vi "Midi_SerialComm.vi"(6 "CtrlC":bool, 8 "error in (no error)":errorcluster, 9 "wait for":string, 10 "To send":string, 11 "hub":string) -> (0 "error out":errorcluster, 2 "read":string)   [LabVIEW 2022 SP3]
panel:
  out "guess":string
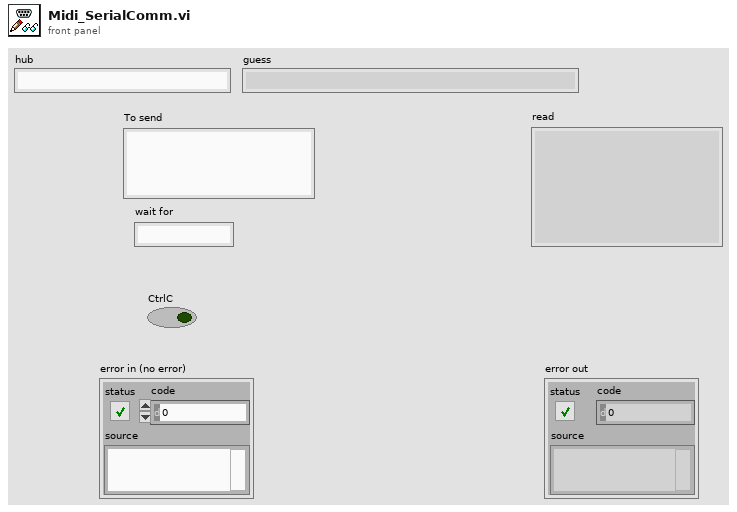
[diagram p1: front panel]
types:
  T1 = typedef "PythonCtrl.ctl" = cluster{"session":refnum<k35>, "PyPath":path, "Processor":T2, "Port":string, "version":string}
  T2 = typedef "Processors.ctl" = enum16{"SPIKE", "Pi", "Pi_ssh", "OpenMV", "Dunio"}
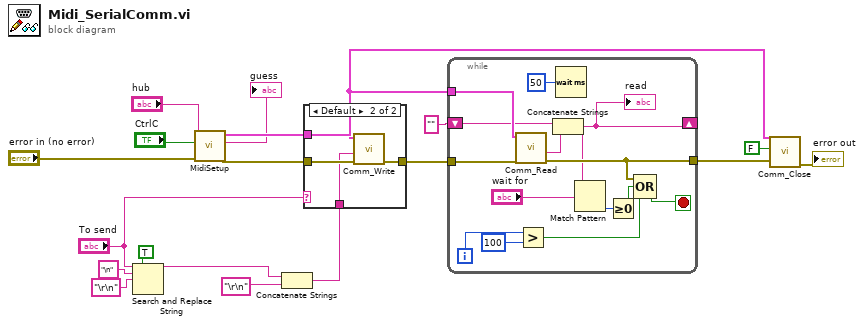
[diagram p0: block diagram]
diagram:
  n1 = Search and Replace String(replace all?=TRUE ("replace all? (F)"), input string="To send", search string="\n" ("function name"), replace string="\r\n" ("function name")) -> (result string=w6:string)  [unwired: 4 in, 3 out]
  n2 = call "MidiSetup.vi"("error in (no error)"="error in (no error)", "CtrlC"="CtrlC", "hub"="hub") -> ("error out"=w17:errorcluster, "guess"=→"guess":string, "Python"=w15:T1)  [unwired: 6 in]
  n3 = Concatenate Strings(w6, "\r\n" ("function name")) -> (w11:string)
  n4 = case shown="Default" "To send" {
    tunnel: w17 -> [w19 w23]
    tunnel: [w19 w22] -> w16
    tunnel: w15 -> [_ w21]
    tunnel: w11 -> [_ w20]
    frame "" {
    }
    frame Default {
      n5 = call "Comm_Write.vi"("error in (no error)"=w23, "Text to write"=w20, "Python"=w21) -> ("error out"=w22:errorcluster)  [unwired: 7 in, 1 out]
    }
  }
  n6 = while {
    tunnel: w16 -> [w37]
    tunnel: w15 -> [w36]
    tunnel: [w30] -> w14
    shift-right: [w27] -> _
    shift-left: "" -> [w34]
    i -> [w26]
    stop <- w29 stop-if-true
    n7 = call "Comm_Read.vi"("error in (no error)"=w37, "Python"=w36) -> ("error out"=w30:errorcluster, "Text read"=w35:string)  [unwired: 8 in]
    n8 = Greater?(x=w26, y=100) -> (0:w24:bool)
    n9 = Concatenate Strings(w34, w35) -> (w27:string)
    "read" <- w27
    n10 = Wait (ms)(milliseconds to wait=u32 50) -> ()  [unwired: 1 out]
    n11 = Match Pattern(string=w27, regular expression="wait for") -> (offset past match=w32:i32)  [unwired: 1 in, 3 out]
    n12 = Greater Or Equal To 0?(x=w32) -> (x >= 0?=w31:bool)
    n13 = Compound Arithmetic op=OR(w30, w31, w24) -> (w29:bool)
  }
  n14 = call "Comm_Close.vi"("error in (no error)"=w14, "Show Err?"=FALSE, "Python in"=w15) -> ("error out"=→"error out":errorcluster)  [unwired: 7 in, 1 out]
